vi "select random file.vi"(11 "Ring":u16) -> (1 "element":string, 2 "size(s)":i32, 3 "filenames":string[](array[string]), 4 "32bit integer":i32, 5 "appended path":path, 6 "all rows":i64[][](array[numeric]), 7 "all rows 2":i64[][](array[numeric]))   [LabVIEW 2021]
uses:
  <vilib>/Utility/file.llb/Read Delimited Spreadsheet (I64).vi
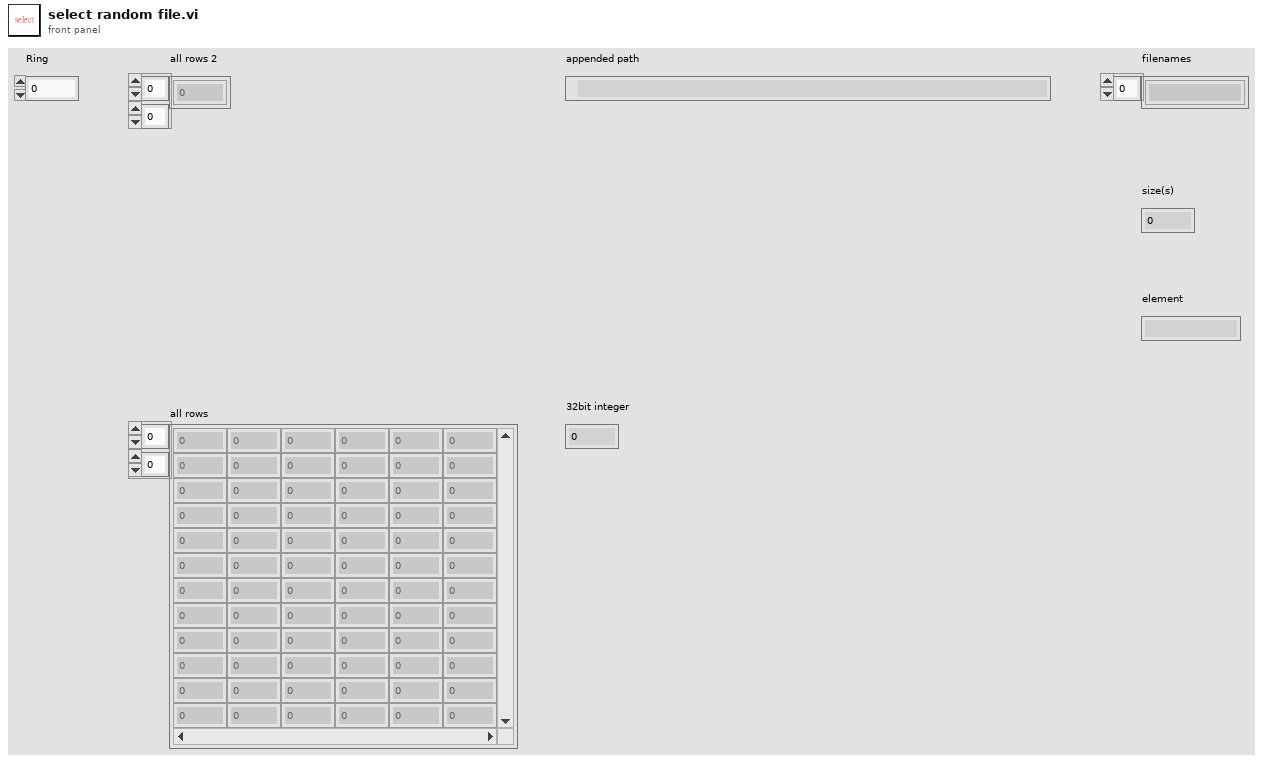
[diagram p1: front panel]
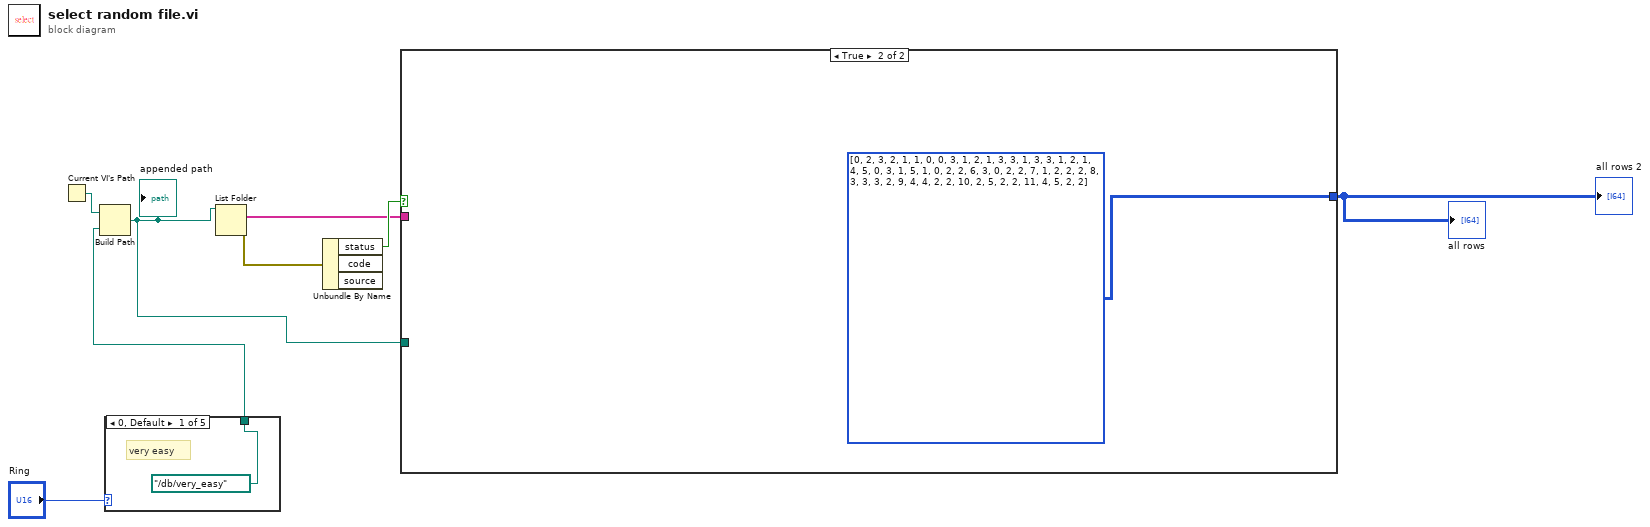
[diagram p0: block diagram]
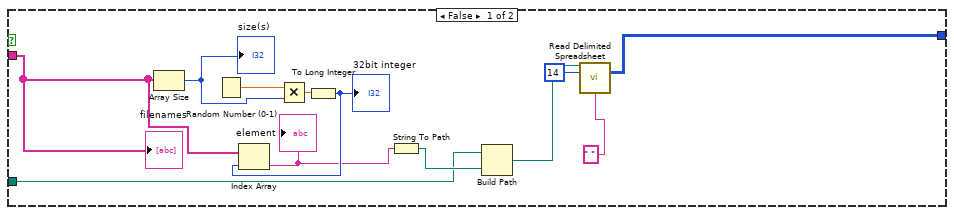
[diagram p2: hidden frame]
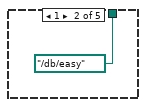
[diagram p3: hidden frame]
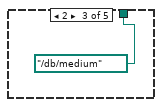
[diagram p4: hidden frame]
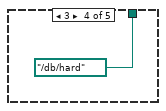
[diagram p5: hidden frame]
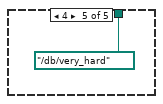
[diagram p6: hidden frame]
diagram:
  n1 = Current VI's Path() -> (path=w7:path)
  n2 = case shown="0, Default" "Ring" {
    tunnel: [path "../db/very_easy" path "../db/easy" path "../db/medium" path "../db/hard" path "../db/very_hard"] -> w8
    frame 0, Default {
      # "very easy"
    }
    frame 1 {
    }
    frame 2 {
    }
    frame 3 {
    }
    frame 4 {
    }
  }
  n3 = Build Path(base path=w7, name or relative path=w8) -> (appended path=w3:path)
  "appended path" <- w3
  n4 = List Folder(path=w3) -> (filenames=w2:string[], error out=w5:errorcluster)  [unwired: 3 in, 2 out]
  n5 = Unbundle By Name(w5) -> ("status"=w4:bool)  [unwired: 2 out]
  n6 = case shown="True" w4 {
    tunnel: w3 -> [w16 _]
    tunnel: w2 -> [w15 _]
    tunnel: [w14 i32[][] [[0, 2, 3, 2, 1], [1, 0, 0, 3, 1], [2, 1, 3, 3, 1], [3, 3, 1, 2, 1], [4, 5, 0, 3, 1], [5, 1, 0, 2, 2], [6, 3, 0, 2, 2], [7, 1, 2, 2, 2], [8, 3, 3, 3, 2], [9, 4, 4, 2, 2], [10, 2, 5, 2, 2], [11, 4, 5, 2, 2]]] -> w1
    frame False {
      n7 = Array Size(array=w15) -> (size(s)=w24:i32)
      "size(s)" <- w24
      n8 = Random Number (0-1)() -> (number: 0 to 1=w23:dbl)
      n9 = Multiply(x=w23, y=w24) -> (x*y=w25:dbl)
      n10 = To Long Integer(number=w25) -> (32bit integer=w22:i32)
      "32bit integer" <- w22
      n11 = Index Array(array=w15, index=w22) -> (element=w21:string)
      "element" <- w21
      n12 = String To Path(string=w21) -> (path=w20:path)
      n13 = Build Path(base path=w16, name or relative path=w20) -> (appended path=w19:path)
      n14 = call-poly <vilib>:"Read Delimited Spreadsheet.vi"("file path (dialog if empty)"=w19, "number of rows (all:-1)"=14, "delimiter (\\t)"=" " ("delimiter (\\t)")) -> ("all rows"=w14:i64[][])  [unwired: 7 in, 5 out]
      "filenames" <- w15
    }
    frame True {
    }
  }
  "all rows" <- w1
  "all rows 2" <- w1
